vi "UpdateMouse.vi"(8 "error in (no error)":errorcluster, 11 "Input in":refnum<class "Input.lvclass">) -> (0 "error out":errorcluster, 3 "Input out":refnum<class "Input.lvclass">)   [LabVIEW 2015, in "Input.lvclass"]
uses:
  Input.lvclass
  Mouse State.ctl
  Input.lvclass/Input.ctl
  <vilib>/Utility/inputDevices.llb/mouseAcquire.vi
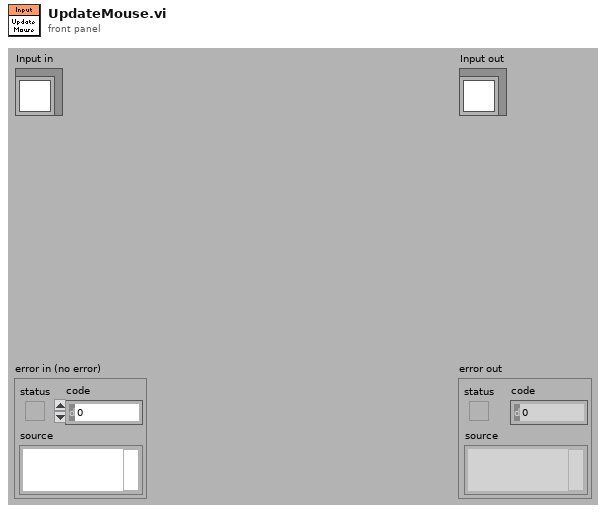
[diagram p1: front panel]
types:
  T1 = typedef "Input.lvclass/Mouse State.ctl" = cluster{"Movement":cluster{"X":i32, "Y":i32, "Scrolling":i32}, "Buttons":cluster{"Button1":bool, "Button2":bool, "Button3":bool, "Button4":bool}}
  T2 = cluster{"Horizontal":i32, "Vertical":i32, "Scrolling":i32}
  T3 = cluster{"button 1":bool, "button 2":bool, "button 3":bool, "button 4":bool}
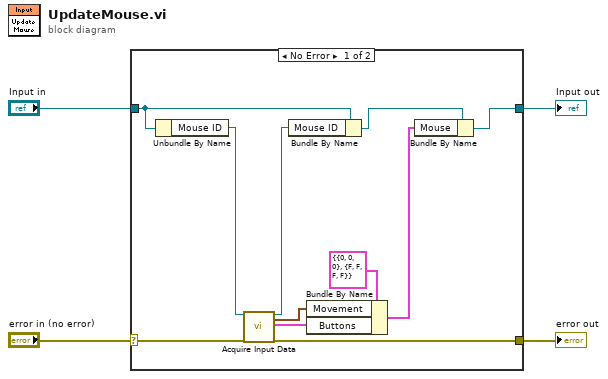
[diagram p0: block diagram]
diagram:
  n1 = case shown="No Error" "error in (no error)" {
    selector: "error in (no error)" -> [w10 w17]
    tunnel: [w5 w17] -> w3
    tunnel: [w7 w16] -> w1
    tunnel: "Input in" -> [w11 w16]
    frame No Error {
      n2 = Unbundle By Name(w11) -> ("Mouse ID"=w15:refnum<k1>)
      n3 = call-poly <vilib>:"Acquire Input Data.vi"("device ID"=w15, "error in (no error)"=w10) -> ("device ID"=w12:refnum<k1>, "axis info"=w14:T2, "button info"=w13:T3, "error out"=w5:errorcluster)  [unwired: 14 in]
      n4 = Bundle By Name(cluster=w11, "Mouse ID"=w12) -> (w8:refnum<class "Input.lvclass">)
      n5 = Bundle By Name(cluster=T1 {"Movement"={"X"=0, "Y"=0, "Scrolling"=0}, "Buttons"={"Button1"=FALSE, "Button2"=FALSE, "Button3"=FALSE, "Button4"=FALSE}} ("Mouse State"), "Movement"=w14, "Buttons"=w13) -> (w6:T1)
      n6 = Bundle By Name(cluster=w8, "Mouse"=w6) -> (w7:refnum<class "Input.lvclass">)
    }
    frame Error {
    }
  }
  "error out" <- w3
  "Input out" <- w1
